vi "WT500 Integration Conditional Start.vi"(8 "error in (no error)":errorcluster, 11 "VISA Refnum in":refnum<visa-resource-name>) -> (0 "error out":errorcluster, 3 "VISA Refnum out":refnum<visa-resource-name>)   [LabVIEW 2012]
doc: "This VI query the Yokogawa WT500 to find out if it is integrating. If it is NOT, it will reset and start ingration."
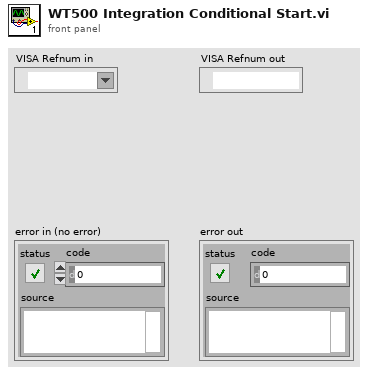
[diagram p1: front panel]
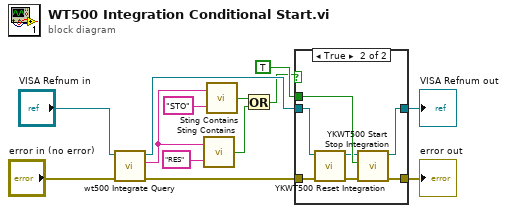
[diagram p0: block diagram]
diagram:
  n1 = call "wt500 Integrate Query.vi"("error in (no error)"="error in (no error)", "VISA resource name"="VISA Refnum in") -> ("error out"=w10:errorcluster, "read buffer"=w5:string, "VISA resource name out"=w9:refnum<visa-resource-name>)  [unwired: 7 in]
  n2 = call "Sting Contains.vi"("Expression to evaluate"="RES", "Input String"=w5) -> ("Boolean"=w2:bool)
  n3 = call "Sting Contains.vi"("Expression to evaluate"="STO", "Input String"=w5) -> ("Boolean"=w3:bool)
  n4 = Or(x=w3, y=w2) -> (x .or. y?=w1:bool)
  n5 = case shown="True" w1 {
    tunnel: w9 -> [w15 w21]
    tunnel: w10 -> [w14 w20]
    tunnel: [w15 w17] -> w11
    tunnel: [w14 w16] -> w12
    tunnel: TRUE ("Start/Stop (False: Stop)") -> [_ w22]
    frame False {
    }
    frame True {
      n6 = call <instrlib>:"YKWT500 Reset Integration.vi"("error in (no error)"=w20, "VISA resource name"=w21) -> ("error out"=w18:errorcluster, "VISA resource name out"=w19:refnum<visa-resource-name>)  [unwired: 8 in]
      n7 = call <instrlib>:"YKWT500 Start Stop Integration.vi"("error in (no error)"=w18, "Start/Stop (False: Stop)"=w22, "VISA resource name"=w19) -> ("error out"=w16:errorcluster, "VISA resource name out"=w17:refnum<visa-resource-name>)  [unwired: 7 in]
    }
  }
  "error out" <- w12
  "VISA Refnum out" <- w11
